vi "1_basic.vi"() -> ()   [LabVIEW 2024]
panel:
  in  "stop":bool
  in  "input string":string
  out "result":string
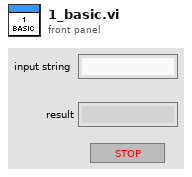
[diagram p1: front panel]
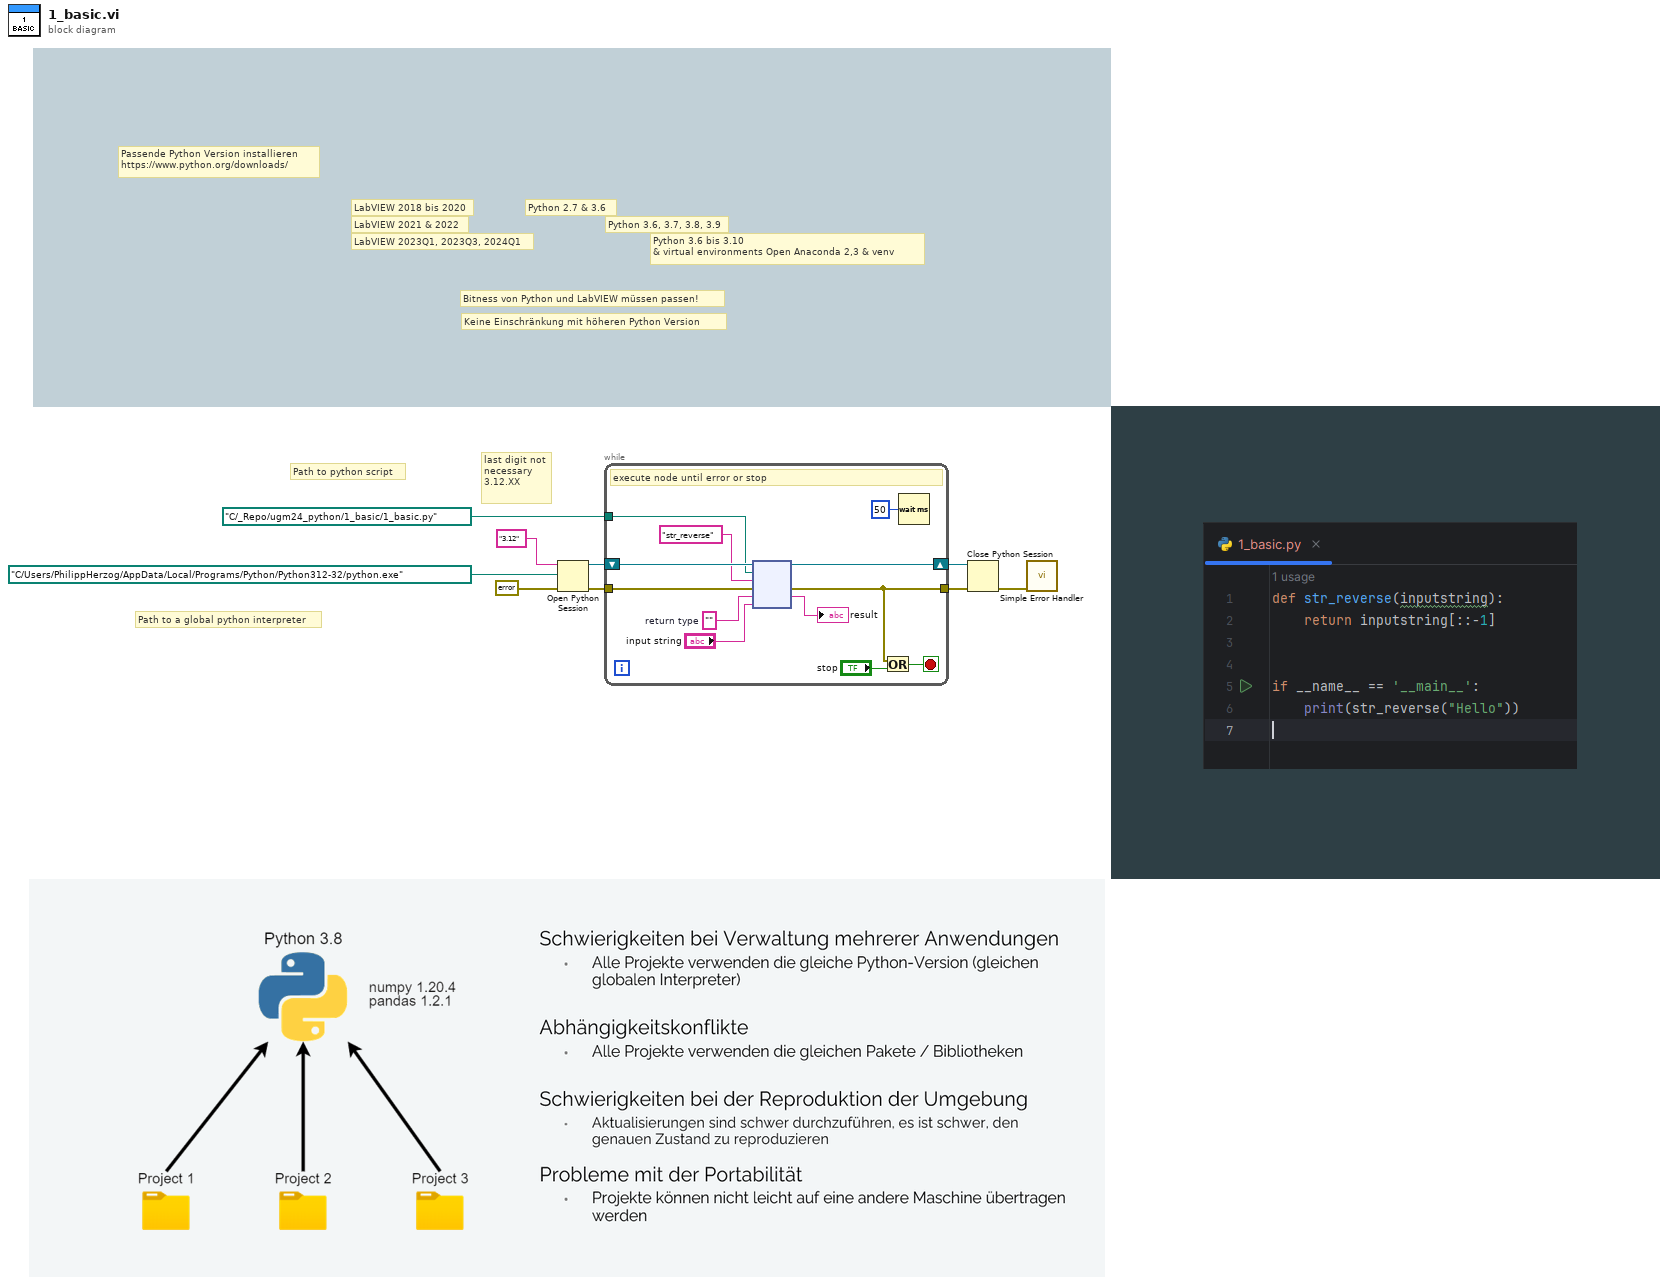
[diagram p0: block diagram]
diagram:
  # "Keine Einschränkung mit höheren Python Version"
  # "Passende Python Version installieren\nhttps://www.python.org/downloads/"
  # "LabVIEW 2023Q1, 2023Q3, 2024Q1"
  # "LabVIEW 2021 & 2022"
  # "LabVIEW 2018 bis 2020"
  # "Python 3.6 bis 3.10\n& virtual environments Open Anaconda 2,3 & venv"
  # "Python 3.6, 3.7, 3.8, 3.9"
  # "Python 2.7 & 3.6"
  # "last digit not\nnecessary\n3.12.XX"
  # "Path to a global python interpreter"
  # "Path to python script"
  # "Bitness von Python und LabVIEW müssen passen!"
  n1 = Open Python Session(python version="3.12" ("Python version"), python path=path "C:/Users/PhilippHerzog/AppData/Local/Programs/Python/Python312-32/python.exe" ("Python path"), 3:errorcluster {"status"=FALSE, "code"=0, "source"=""} ("error in (no error)")) -> (session out=w6:refnum<k35>, error out=w9:errorcluster)
  n2 = while {
    tunnel: w9 -> [w21]
    tunnel: path "C:/_Repo/ugm24_python/1_basic/1_basic.py" ("Path") -> [w19]
    tunnel: [w13] -> w4
    shift-right: [w12] -> w3
    shift-left: w6 -> [w20]
    stop <- w15 stop-if-true
    w10 = ""  # return type
    # "execute node until error or stop"
    n3 = node(w20, w19, "str_reverse" ("function name"), w21, w10, "input string") -> (w12:refnum<k35>, w13:errorcluster, →"result":string)  [unwired: 1 in, 2 out]
    n4 = Or(x=w13, y="stop") -> (x .or. y?=w15:bool)
    n5 = Wait (ms)(milliseconds to wait=u32 50) -> ()  [unwired: 1 out]
  }
  n6 = Close Python Session(session in=w3, error in=w4) -> (11:w2:errorcluster)
  n7 = call <vilib>:"Simple Error Handler.vi"("error in (no error)"=w2) -> ()  [unwired: 4 in, 5 out]
